vi "Wait for Acquisition Complete.vi"(8 "error in (no error)":errorcluster {"code" format="%.0x"}, 10 "Maximum Time (10000 ms)":u32=10000, 11 "VISA Resource Name":refnum<visa-resource-name>) -> (0 "error out":errorcluster {"code" format="%.0x"}, 3 "VISA Resource Name Out":refnum<visa-resource-name>)   [LabVIEW 2010, in "Tektronix TDS 3000 Series.lvlib"]
doc: "Waits for the current waveform acquisition to finish. This VI should be called after <B>Initiate VI</B> and before <B>Fetch Waveform VI</B>.\n\n<B>Note:</B> \n\nThis VI should only be used when the scope is in single acquisition mode, otherwise a timeout error will be thrown. Set the Continuous Acquisition control to False in <B>Configure Initiate Continous VI</B> to ensure single-sequence acquisition mode is enabled before calling this VI."
uses:
  <instrlib>/Tektronix TDS 3000 Series/Tektronix TDS 3000 Series.lvlib
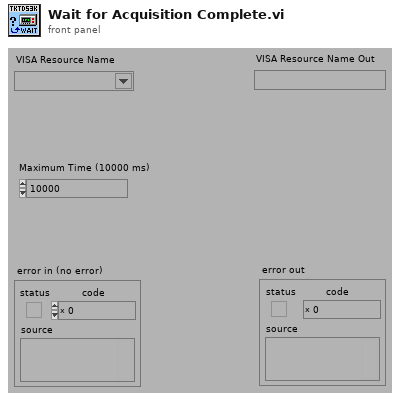
[diagram p1: front panel]
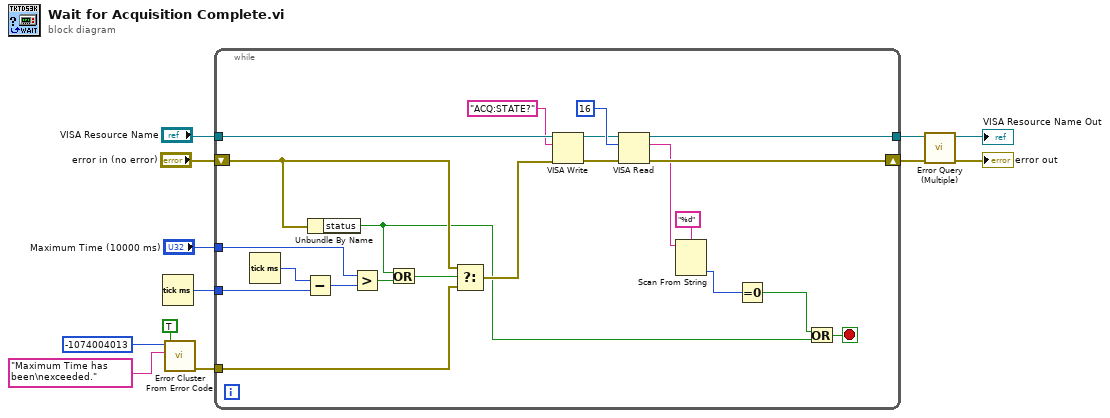
[diagram p0: block diagram]
diagram:
  n1 = Tick Count (ms)() -> (millisecond timer value=w12:u32)
  n2 = call <vilib>:"Error Cluster From Error Code.vi"("show call chain? (False)"=TRUE, "error message (\"\")"="Maximum Time has been\nexceeded." ("error message (\"\")"), "error code (0)"=-1074004013) -> ("error out"=w8:errorcluster)  [unwired: 6 in]
  n3 = while {
    tunnel: [w33] -> w4
    tunnel: "VISA Resource Name" -> [w32]
    tunnel: "Maximum Time (10000 ms)" -> [w28]
    tunnel: w12 -> [w29]
    tunnel: w8 -> [w24]
    shift-right: [w34] -> w3
    shift-left: "error in (no error)" -> [w25]
    stop <- w22 stop-if-true
    n4 = Tick Count (ms)() -> (millisecond timer value=w31:u32)
    n5 = Subtract(x=w31, y=w29) -> (x-y=w30:u32)
    n6 = Unbundle By Name(w25) -> ("status"=w21:bool)
    n7 = Greater?(x=w28, y=w30) -> (0:w27:bool)
    n8 = Or(x=w21, y=w27) -> (x .or. y?=w26:bool)
    n9 = Select(t=w25, s=w26, f=w24) -> (s? t:f=w23:errorcluster)
    n10 = VISA Write(VISA resource name=w32, write buffer="ACQ:STATE?", error in (no error)=w23) -> (VISA resource name out=w15:refnum<visa-resource-name>, error out=w16:errorcluster)  [unwired: 1 out]
    n11 = VISA Read(VISA resource name=w15, byte count=u32 16, error in (no error)=w16) -> (VISA resource name out=w33:refnum<visa-resource-name>, read buffer=w20:string, error out=w34:errorcluster)  [unwired: 1 out]
    n12 = Scan From String(format string="%d", input string=w20) -> (output 1=w14:i32)  [unwired: 3 in, 3 out]
    n13 = Equal To 0?(x=w14) -> (x = 0?=w13:bool)
    n14 = Or(x=w13, y=w21) -> (x .or. y?=w22:bool)
  }
  n15 = call <instrlib>:"Error Query (Multiple).vi"("error in (no error)"=w3, "VISA Resource Name"=w4) -> ("error out"=→"error out":errorcluster, "VISA Resource Name Out"=→"VISA Resource Name Out":refnum<visa-resource-name>)  [unwired: 6 in, 2 out]
